vi "SeCrTs-Data.vi"(8 "error in (no error)":errorcluster, 11 "Data FIFO Ref":T1) -> (0 "error out":errorcluster, 3 "data":string)   [LabVIEW 2022 SP3]
uses:
  RT Controls/SeCrTs-Data FIFO.ctl
panel:
  out "# elements in queue 6":i32
  out "# elements in queue 5":i32
  out "# elements in queue 4":i32
  out "# elements in queue 3":i32
  out "# elements in queue 2":i32
  out "# elements in queue":i32
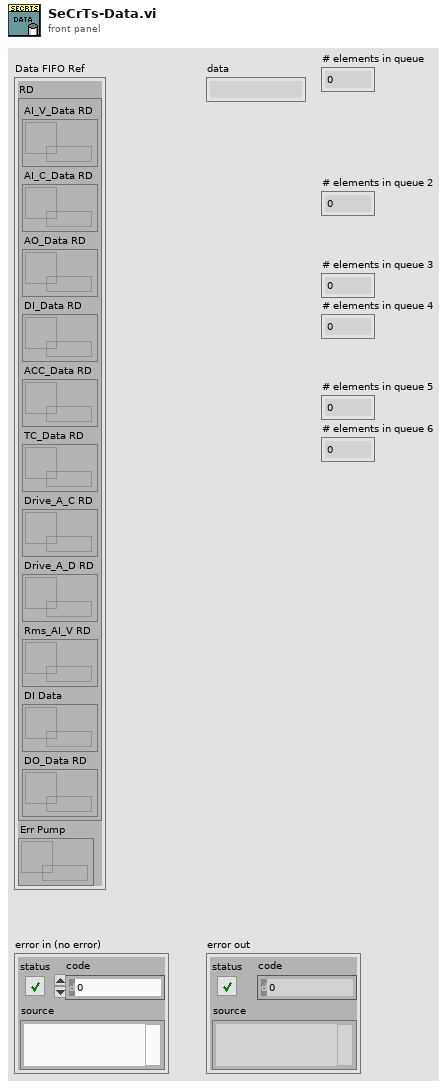
[diagram p1: front panel]
types:
  T1 = typedef "SeCrTs-Data FIFO.ctl" = cluster{"RD":cluster{"AI_V_Data RD":refnum<queue>, "AI_C_Data RD":refnum<queue>, "AO_Data RD":refnum<queue>, "DI_Data RD":refnum<queue>, "ACC_Data RD":refnum<queue>, "TC_Data RD":refnum<queue>, "Drive_A_C RD":refnum<queue>, "Drive_A_D RD":refnum<queue>, "Rms_AI_V RD":refnum<queue>, "DI Data":refnum<queue>, "DO_Data RD":refnum<queue>}, "Err Pump":refnum<queue>}
  T2 = cluster{"AI_V_Data":waveform(dbl)[][], "AI_C_Data":waveform(dbl)[][], "AO_Data":waveform(dbl)[][], "DO_Data":waveform(dbl)[][], "DI_Data":digitalwaveform[][], "ACC_Data":waveform(dbl)[][], "TC Data":waveform(dbl)[][], "Drive_A_C":waveform(dbl)[][], "Drive_A_D":waveform(dbl)[][], "AI_V Rms":waveform(dbl)[][], "Drive":cluster{"Drive_Health":bool, "Drive_Frequency":u32, "Drive_Status":bool, "Drive_RPM":u32, "Drive_Direction":bool, "Acceleration state":bool, "Steady state":bool, "Deceleration state":bool, "Drive_Enable":bool, "Drive set_RPM":dbl}}
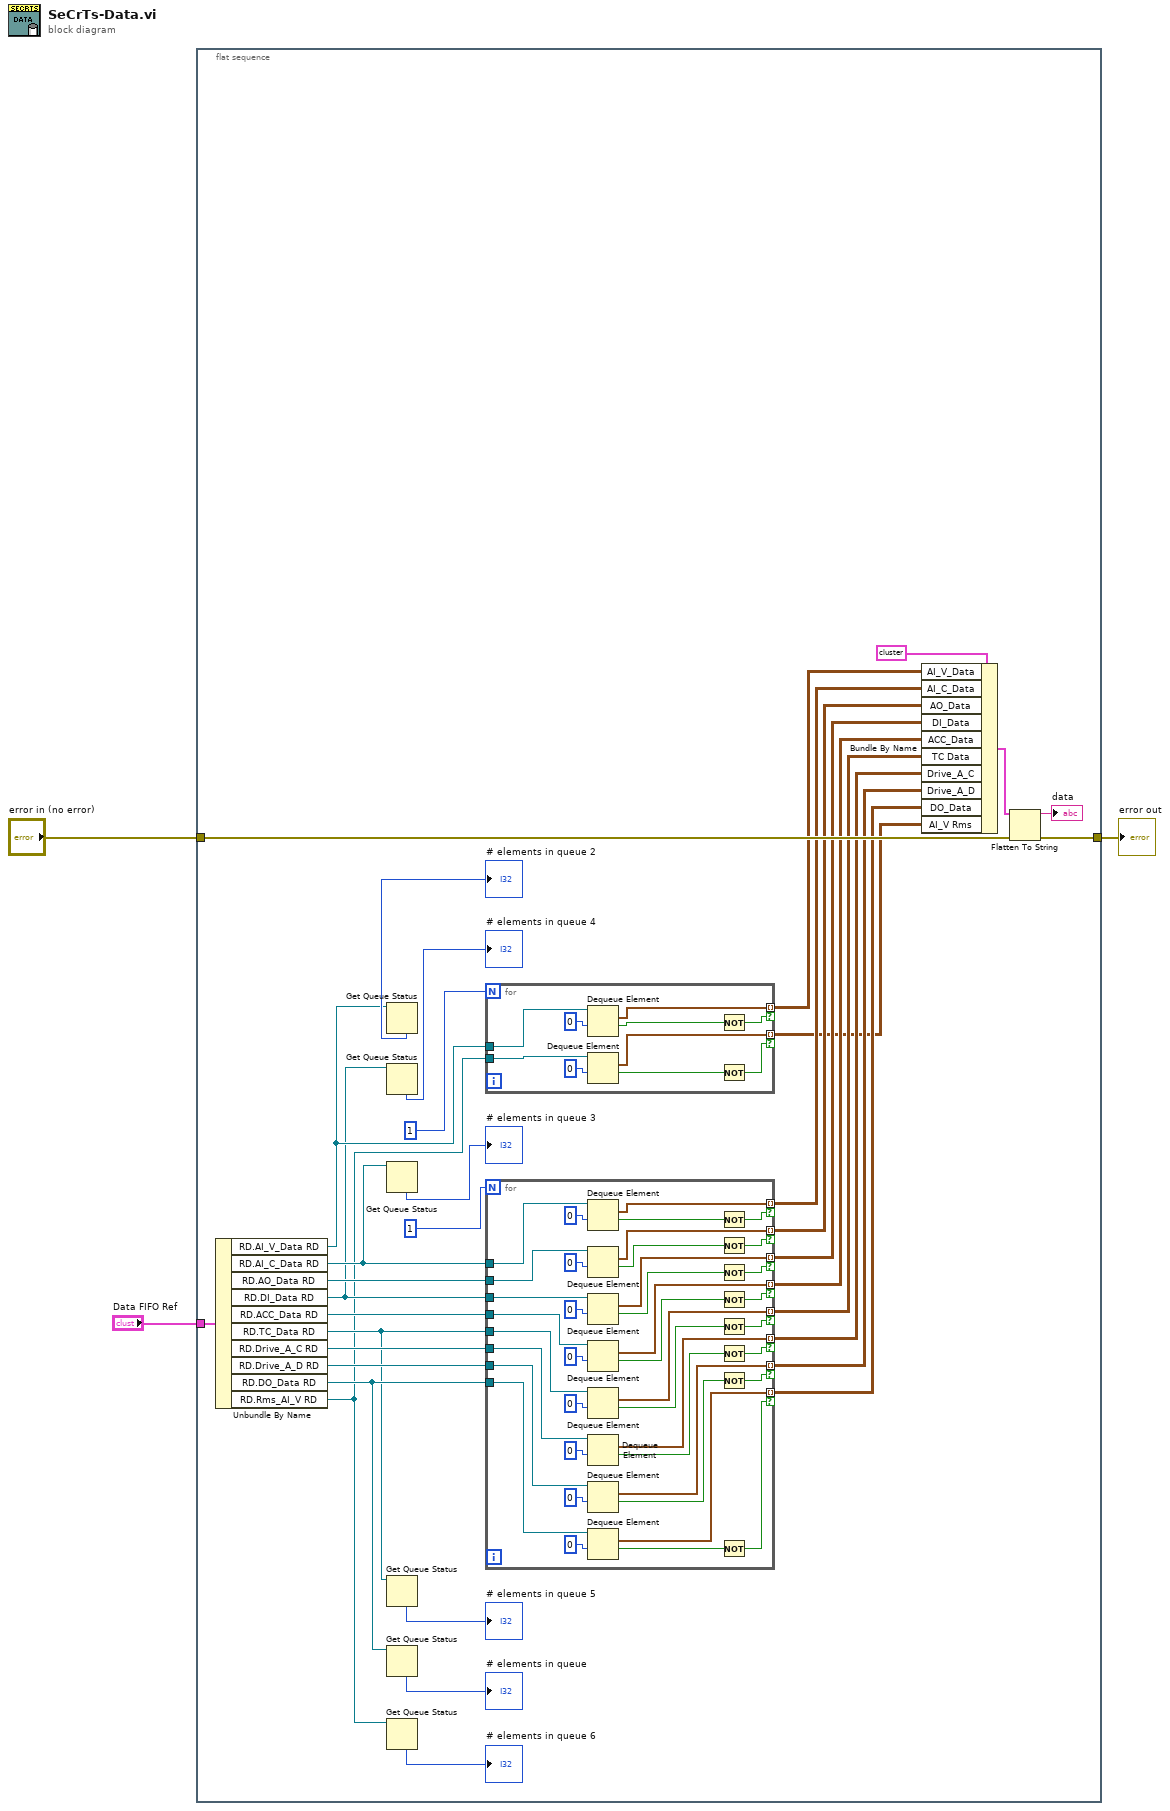
[diagram p0: block diagram]
diagram:
  n1 = flat-sequence {
    tunnel: "Data FIFO Ref" -> [w37]
    tunnel: "error in (no error)" -> [w35]
    tunnel: [w34] -> w1
    frame #0 {
      n2 = Unbundle By Name(w37) -> ("RD.AI_V_Data RD"=w9:refnum<queue>, "RD.AI_C_Data RD"=w8:refnum<queue>, "RD.AO_Data RD"=w32:refnum<queue>, "RD.DI_Data RD"=w7:refnum<queue>, "RD.ACC_Data RD"=w31:refnum<queue>, "RD.TC_Data RD"=w10:refnum<queue>, "RD.Drive_A_C RD"=w30:refnum<queue>, "RD.Drive_A_D RD"=w29:refnum<queue>, "RD.DO_Data RD"=w16:refnum<queue>, "RD.Rms_AI_V RD"=w5:refnum<queue>)
      n3 = Get Queue Status(queue=w9) -> (# elements in queue=→"# elements in queue 2":i32)  [unwired: 2 in, 7 out]
      n4 = Get Queue Status(queue=w7) -> (# elements in queue=→"# elements in queue 4":i32)  [unwired: 2 in, 7 out]
      n5 = Get Queue Status(queue=w8) -> (# elements in queue=→"# elements in queue 3":i32)  [unwired: 2 in, 7 out]
      n6 = Get Queue Status(queue=w10) -> (# elements in queue=→"# elements in queue 5":i32)  [unwired: 2 in, 7 out]
      n7 = Get Queue Status(queue=w16) -> (# elements in queue=→"# elements in queue":i32)  [unwired: 2 in, 7 out]
      n8 = Get Queue Status(queue=w5) -> (# elements in queue=→"# elements in queue 6":i32)  [unwired: 2 in, 7 out]
      n9 = for {
        N: 1 -> [_]
        tunnel: w9 -> [w45]
        tunnel: [w44] -> w20 mode=indexing if=w43
        tunnel: w5 -> [w42]
        tunnel: [w39] -> w4 mode=indexing if=w38
        n10 = Dequeue Element(queue=w45, timeout in ms (-1)=0) -> (element=w44:waveform(dbl)[], timed out?=w46:bool)  [unwired: 1 in, 2 out]
        n11 = Dequeue Element(queue=w42, timeout in ms (-1)=0) -> (element=w39:waveform(dbl)[], timed out?=w40:bool)  [unwired: 1 in, 2 out]
        n12 = Not(x=w46) -> (.not. x?=w43:bool)
        n13 = Not(x=w40) -> (.not. x?=w38:bool)
      }
      n14 = for {
        N: 1 -> [_]
        tunnel: w8 -> [w87]
        tunnel: w32 -> [w86]
        tunnel: w7 -> [w85]
        tunnel: w31 -> [w84]
        tunnel: w10 -> [w83]
        tunnel: w30 -> [w82]
        tunnel: w29 -> [w81]
        tunnel: w16 -> [w51]
        tunnel: [w80] -> w28 mode=indexing if=w61
        tunnel: [w79] -> w27 mode=indexing if=w60
        tunnel: [w78] -> w26 mode=indexing if=w59
        tunnel: [w77] -> w25 mode=indexing if=w58
        tunnel: [w76] -> w24 mode=indexing if=w57
        tunnel: [w75] -> w23 mode=indexing if=w56
        tunnel: [w74] -> w22 mode=indexing if=w53
        tunnel: [w50] -> w18 mode=indexing if=w49
        n15 = Dequeue Element(queue=w87, timeout in ms (-1)=0) -> (element=w80:waveform(dbl)[], timed out?=w62:bool)  [unwired: 1 in, 2 out]
        n16 = Dequeue Element(queue=w86, timeout in ms (-1)=0) -> (element=w79:waveform(dbl)[], timed out?=w64:bool)  [unwired: 1 in, 2 out]
        n17 = Dequeue Element(queue=w85, timeout in ms (-1)=0) -> (element=w78:digitalwaveform[], timed out?=w66:bool)  [unwired: 1 in, 2 out]
        n18 = Dequeue Element(queue=w84, timeout in ms (-1)=0) -> (element=w77:waveform(dbl)[], timed out?=w68:bool)  [unwired: 1 in, 2 out]
        n19 = Dequeue Element(queue=w83, timeout in ms (-1)=0) -> (element=w76:waveform(dbl)[], timed out?=w70:bool)  [unwired: 1 in, 2 out]
        n20 = Dequeue Element(queue=w82, timeout in ms (-1)=0) -> (element=w75:waveform(dbl)[], timed out?=w72:bool)  [unwired: 1 in, 2 out]
        n21 = Dequeue Element(queue=w81, timeout in ms (-1)=0) -> (element=w74:waveform(dbl)[], timed out?=w54:bool)  [unwired: 1 in, 2 out]
        n22 = Dequeue Element(queue=w51, timeout in ms (-1)=0) -> (element=w50:waveform(dbl)[], timed out?=w48:bool)  [unwired: 1 in, 2 out]
        n23 = Not(x=w62) -> (.not. x?=w61:bool)
        n24 = Not(x=w64) -> (.not. x?=w60:bool)
        n25 = Not(x=w66) -> (.not. x?=w59:bool)
        n26 = Not(x=w68) -> (.not. x?=w58:bool)
        n27 = Not(x=w70) -> (.not. x?=w57:bool)
        n28 = Not(x=w72) -> (.not. x?=w56:bool)
        n29 = Not(x=w54) -> (.not. x?=w53:bool)
        n30 = Not(x=w48) -> (.not. x?=w49:bool)
      }
      n31 = Bundle By Name(cluster=T2 data[101863B] ("data out"), "AI_V_Data"=w20, "AI_C_Data"=w28, "AO_Data"=w27, "DI_Data"=w26, "ACC_Data"=w25, "TC Data"=w24, "Drive_A_C"=w23, "Drive_A_D"=w22, "DO_Data"=w18, "AI_V Rms"=w4) -> (w33:T2)
      n32 = Flatten To String(anything=w33, error in (no error)=w35) -> (data string=→"data":string, error out=w34:errorcluster)  [unwired: 2 in, 1 out]
    }
  }
  "error out" <- w1
